vi "Process.vi"(8 "error in (no error)":errorcluster, 11 "Execution Profiler In":refnum<class "Execution Profiler.lvclass">) -> (0 "error out":errorcluster, 3 "Execution Profiler Out":refnum<class "Execution Profiler.lvclass">)   [LabVIEW 2020, in "Execution Profiler.lvclass"]
uses:
  Execution Profiler.lvclass
  C:/Git/astemes-lunit/source/Application Framework/Process Classes/Process/Process.lvclass
  Application Framework/Process Classes/Process/Process.lvclass/Process.ctl
  Result Types/Method Result/Method Result.ctl
  Rewrite Project/Result/Status.ctl
  Result Types/Assertion Result/Assertion Result.ctl
  Result Types/Assertion Result/Public/TypeDefs/Assertion Type.ctl
  Result Types/Case Result/Test Case Result.ctl
  Result Types/Suite Results/Test Suite Result.ctl
  Result Types/Assertion Result/Public/TypeDefs/Status.ctl
  Execution Profiler.lvclass/Execution Profiler.ctl
  Helper Classes/Open Test Case Interface/Open Test Case.lvclass
  Application Framework/Process Classes/Process/Public/Accessors/Read Process Name.vi
  <vilib>/Utility/error.llb/Error Cluster From Error Code.vi
  Application Framework/Process Classes/Error Handler/Private/SubVIs/Get Error Queue Name.vi
  <vilib>/ErrorRing/Error Ring.xnode
  Application Framework/Process Classes/Process/Process.lvclass
  Application Framework/Process Classes/Error Handler/Error Handler.lvclass
  Result Types/Assertion Result/Assertion Result.lvlib
  Result Types/Method Result/Method Result.lvlib
  Result Types/Case Result/Test Case Result.lvlib
  Result Types/Suite Results/Test Suite Result.lvlib
  Rewrite Project/Result/Result.lvlib
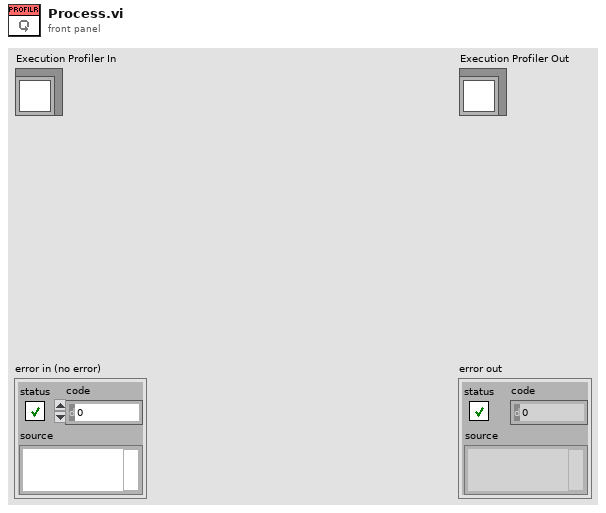
[diagram p1: front panel]
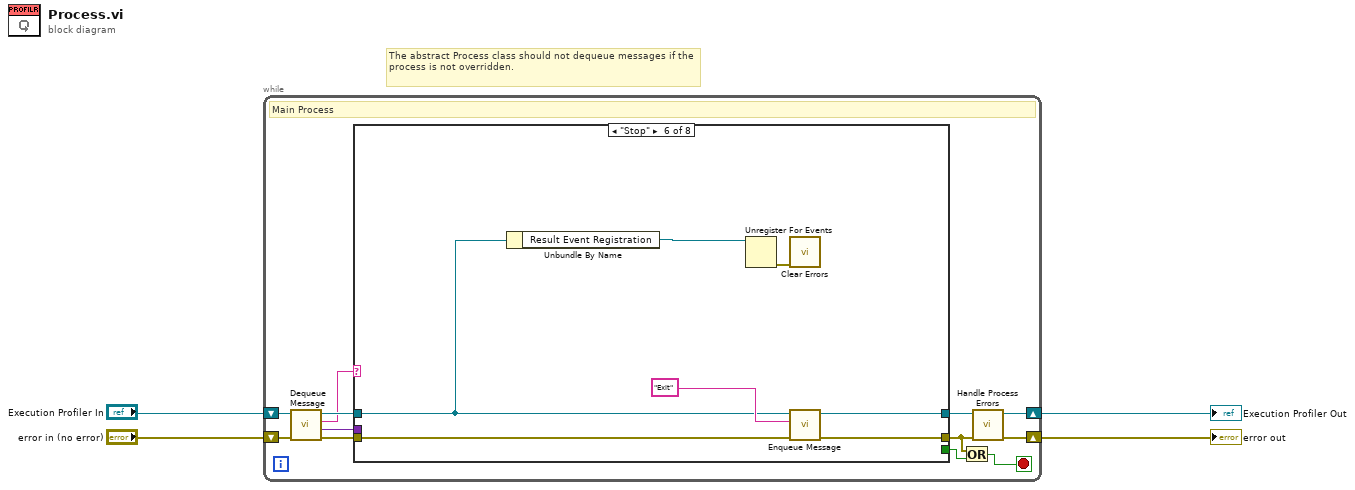
[diagram p0: block diagram]
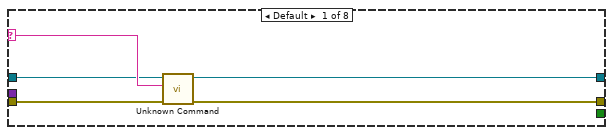
[diagram p2: hidden frame]
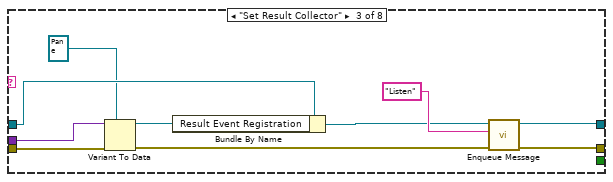
[diagram p4: hidden frame]
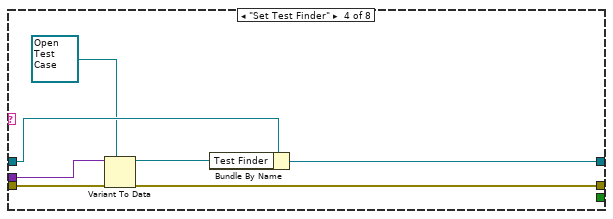
[diagram p5: hidden frame]
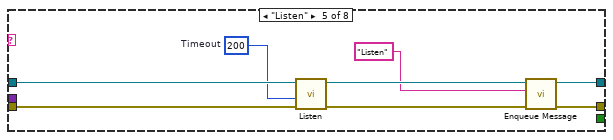
[diagram p6: hidden frame]
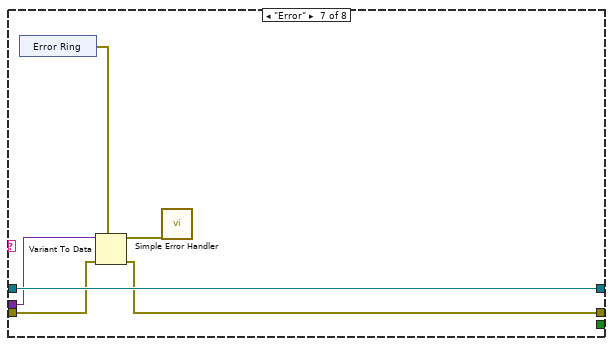
[diagram p7: hidden frame]
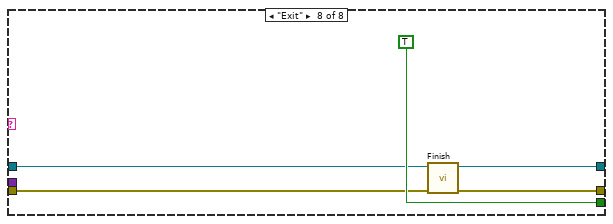
[diagram p8: hidden frame]
diagram:
  # "The abstract Process class should not dequeue messages if the process is not overridden."
  n1 = while {
    shift-right: [w9] -> w4
    shift-left: "error in (no error)" -> [w15]
    shift-right: [w7] -> w3
    shift-left: "Execution Profiler In" -> [w16]
    stop <- w6 stop-if-true
    # "Main Process"
    n2 = call "Dequeue Message.vi"("error in (no error)"=w15, "Process In"=w16) -> ("error out"=w14:errorcluster, "Message Data"=w11:variant, "Message"=w12:string, "Process Out"=w13:refnum<class "Execution Profiler.lvclass">)  [unwired: 6 in]
    n3 = case shown="\"Stop\"" w12 {
      selector: w12 -> [w21 _ _ _ _ _ _ _]
      tunnel: [w18 w23 w26 w35 w47 w53 w57 w64] -> w5
      tunnel: w14 -> [w17 w23 w32 w38 w45 w54 w60 w63]
      tunnel: [w20 w22 w27 w36 w48 w52 w61 w65] -> w8
      tunnel: w13 -> [w19 w22 w31 w37 w46 w51 w61 w66]
      tunnel: w11 -> [_ _ w33 w39 _ _ w59 _]
      tunnel: [_ _ _ _ _ _ _ TRUE] -> w10
      frame Default {
        n4 = call "Unknown Command.vi"("error in (no error)"=w17, "String"=w21, "Process In"=w19) -> ("error out"=w18:errorcluster, "Process Out"=w20:refnum<class "Execution Profiler.lvclass">)  [unwired: 7 in]
      }
      frame "Init" {
      }
      frame "Set Result Collector" {
        n5 = Variant To Data(error in=w32, type=refnum<event-registration> refnum ("Result Events"), Variant=w33) -> (data=w24:refnum<event-registration>, error out=w29:errorcluster)
        n6 = Bundle By Name(cluster=w31, "Result Event Registration"=w24) -> (w28:refnum<class "Execution Profiler.lvclass">)
        n7 = call "Enqueue Message.vi"("error in (no error)"=w29, "Message"="Listen", "Process In"=w28) -> ("error out"=w26:errorcluster, "Process Out"=w27:refnum<class "Execution Profiler.lvclass">)  [unwired: 7 in]
      }
      frame "Set Test Finder" {
        n8 = Variant To Data(error in=w38, type=refnum<class "Open Test Case.lvclass"> refnum ("Open Test Case.lvclass"), Variant=w39) -> (data=w40:refnum<class "Open Test Case.lvclass">, error out=w35:errorcluster)
        n9 = Bundle By Name(cluster=w37, "Test Finder"=w40) -> (w36:refnum<class "Execution Profiler.lvclass">)
      }
      frame "Listen" {
        w42 = 200  # Timeout
        n10 = call "Listen.vi"("error in (no error)"=w45, "Timeout"=w42, "Execution Profiler In"=w46) -> ("error out"=w43:errorcluster, "Execution Profiler Out"=w44:refnum<class "Execution Profiler.lvclass">)  [unwired: 7 in]
        n11 = call "Enqueue Message.vi"("error in (no error)"=w43, "Message"="Listen", "Process In"=w44) -> ("error out"=w47:errorcluster, "Process Out"=w48:refnum<class "Execution Profiler.lvclass">)  [unwired: 7 in]
      }
      frame "Stop" {
        n12 = Unbundle By Name(w51) -> ("Result Event Registration"=w49:refnum<event-registration>)
        n13 = Unregister For Events(event registration refnum=w49) -> (error out=w50:errorcluster)  [unwired: 1 in]
        n14 = call <vilib>:"Clear Errors.vi"("error in (no error)"=w50) -> ()  [unwired: 5 in, 2 out]
        n15 = call "Enqueue Message.vi"("error in (no error)"=w54, "Message"="Exit", "Process In"=w51) -> ("error out"=w53:errorcluster, "Process Out"=w52:refnum<class "Execution Profiler.lvclass">)  [unwired: 7 in]
      }
      frame "Error" {
        n16 = xnode "Error Ring"() -> ("error out"=w58:errorcluster)
        n17 = Variant To Data(error in=w60, type=w58, Variant=w59) -> (data=w56:errorcluster, error out=w57:errorcluster)
        n18 = call <vilib>:"Simple Error Handler.vi"("error in (no error)"=w56) -> ()  [unwired: 4 in, 5 out]
      }
      frame "Exit" {
        n19 = call "Finish.vi"("error in (no error)"=w63, "Process In"=w66) -> ("error out"=w64:errorcluster, "Process Out"=w65:refnum<class "Execution Profiler.lvclass">)  [unwired: 8 in]
      }
    }
    n20 = Or(x=w5, y=w10) -> (x .or. y?=w6:bool)
    n21 = call "Handle Process Errors.vi"("error in (no error)"=w5, "Process In"=w8) -> ("error out"=w9:errorcluster, "Process Out"=w7:refnum<class "Execution Profiler.lvclass">)  [unwired: 8 in]
  }
  "error out" <- w4
  "Execution Profiler Out" <- w3
